vi "RT Loop message processing.vi"(7 "queue processing cycle time":u32=50 min=1 max=500, 8 "error in (no error)":errorcluster, 10 "reserved cycle for lower priority queues":u32=10 min=5 max=100) -> ()   [LabVIEW 2016]
uses:
  Globals/RT Stop.vi
  Globals/queue priority list.vi
  Message Queue/Message Queue.lvlib
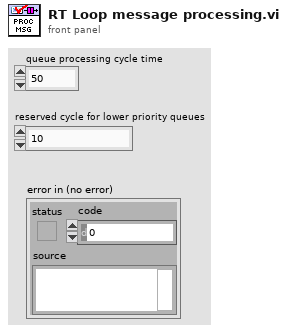
[diagram p1: front panel]
types:
  T1 = typedef "Message Queue.lvlib/queue priority list.ctl" = T2[]
  T2 = typedef "Message Queue.lvlib/queue priority info.ctl" = cluster{"queue name":string, "msg processing func ref":refnum<vi>}
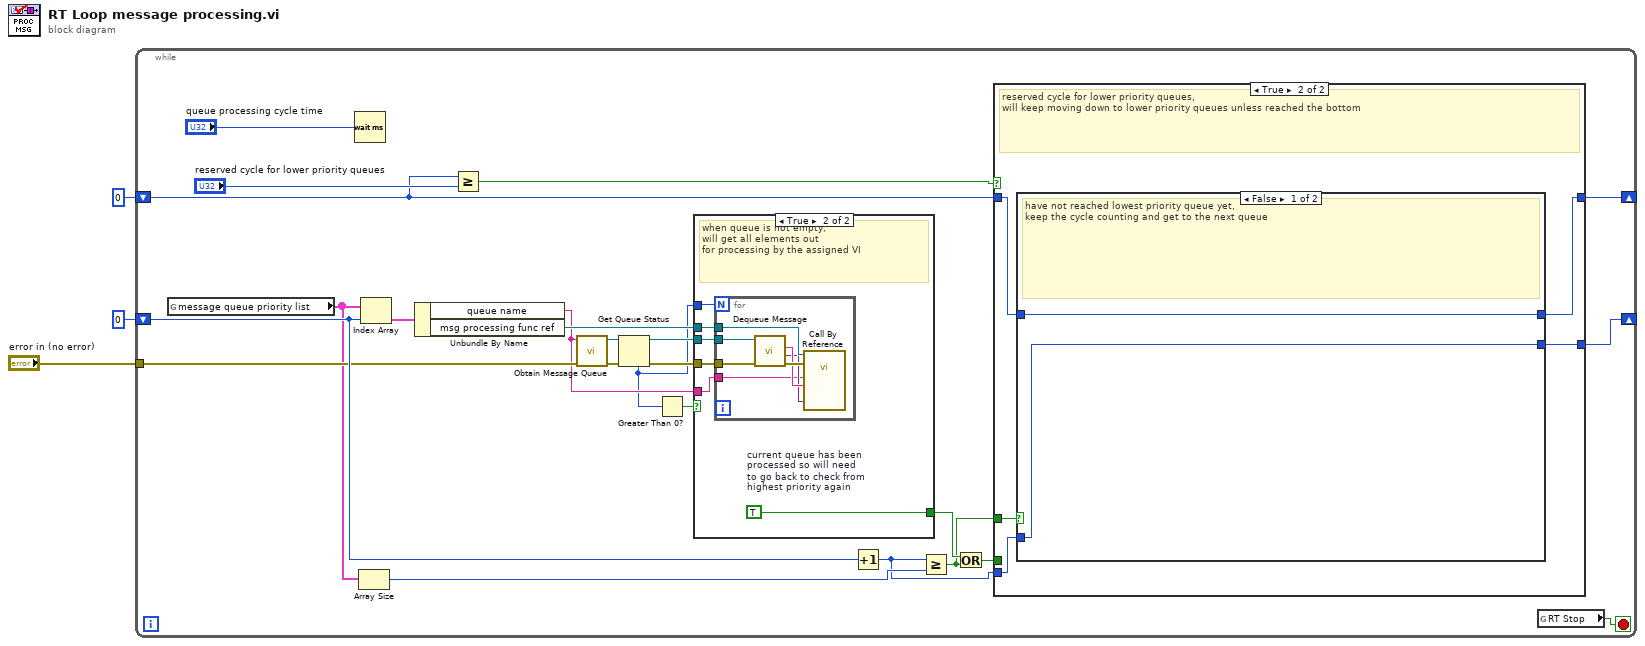
[diagram p0: block diagram]
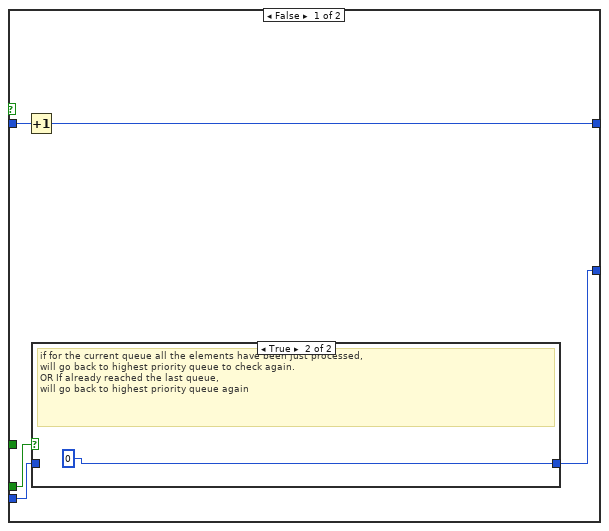
[diagram p2: hidden frame]
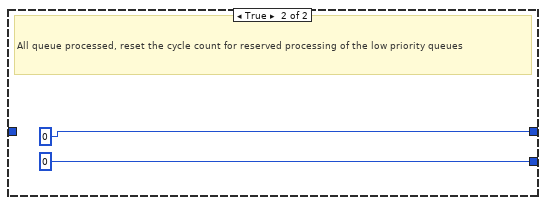
[diagram p4: hidden frame]
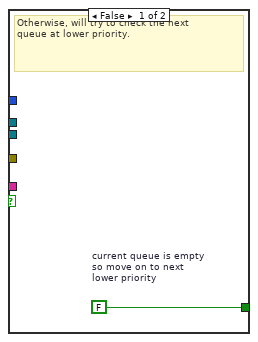
[diagram p5: hidden frame]
diagram:
  n1 = while {
    shift-right: [w24] -> _
    shift-left: 0 -> [w26]
    tunnel: "error in (no error)" -> [w25]
    shift-right: [w5] -> _
    shift-left: u32 0 -> [w6]
    stop <- w27 stop-if-true
    n2 = global read "queue priority list.vi" "message queue priority list"() -> (w16:T1)
    n3 = Wait (ms)(milliseconds to wait="queue processing cycle time") -> ()  [unwired: 1 out]
    n4 = Array Size(array=w16) -> (size(s)=w15:i32)
    n5 = Index Array(array=w16, index=w26) -> (element=w23:T2)
    n6 = Unbundle By Name(w23) -> ("queue name"=w17:string, "msg processing func ref"=w21:refnum<vi>)
    n7 = Greater Or Equal?(x=w6, y="reserved cycle for lower priority queues") -> (x >= y?=w8:bool)
    n8 = call "Obtain Message Queue.vi"("error in (no error)"=w25, "name (unnamed)"=w17) -> ("error out"=w19:errorcluster, "Message Queue"=w22:refnum<queue>)  [unwired: 7 in, 1 out]
    n9 = Get Queue Status(queue=w22, error in (no error)=w19) -> (queue out=w20:refnum<queue>, error out=w18:errorcluster, # elements in queue=w14:i32)  [unwired: 1 in, 5 out]
    n10 = Greater Than 0?(x=w14) -> (x > 0?=w13:bool)
    n11 = case shown="True" w13 {
      tunnel: w21 -> [_ w50]
      tunnel: w20 -> [_ w49]
      tunnel: w18 -> [_ w48]
      tunnel: w17 -> [_ w47]
      tunnel: w14 -> [_ w46]
      tunnel: [w44 w45] -> w11
      frame False {
        w44 = FALSE  # current queue is empty so move on to next lower priority
        # "Otherwise, will try to check the next \nqueue at lower priority."
      }
      frame True {
        w45 = TRUE  # current queue has been processed so will need to go back to check from highest priority again
        # "when queue is not empty,\nwill get all elements out\nfor processing by the assigned VI"
        n12 = for {
          N: w46 -> [_]
          tunnel: w50 -> [w57]
          tunnel: w49 -> [w56]
          tunnel: w48 -> [w55]
          tunnel: w47 -> [w51]
          n13 = call "Dequeue Message.vi"("error in (no error)"=w55, "Message Queue"=w56) -> ("error out"=w54:errorcluster, "Message Data"=w52:variant, "Message"=w53:string)  [unwired: 5 in, 2 out]
          n14 = call-by-ref "?"(reference=w57, error in=w54, "message data"=w52, "message"=w53, "message type"=w51) -> ()  [unwired: 9 in, 2 out]
        }
      }
    }
    n15 = Increment(x=w26) -> (x+1=w9:i32)
    n16 = Greater Or Equal?(x=w9, y=w15) -> (x >= y?=w7:bool)
    n17 = Or(x=w11, y=w7) -> (x .or. y?=w12:bool)
    n18 = case shown="True" w8 {
      tunnel: [w32 w38] -> w24
      tunnel: w12 -> [w31 _]
      tunnel: w9 -> [w30 w37]
      tunnel: w7 -> [_ w39]
      tunnel: w6 -> [w29 w36]
      tunnel: [w28 w35] -> w5
      frame False {
        n19 = Increment(x=w29) -> (x+1=w28:u32)
        n20 = case shown="True" w31 {
          tunnel: w30 -> [w33 _]
          tunnel: [w33 0] -> w32
          frame False {
            # "Otherwise, if the current queue has nothing in it to process, \nand there are lower priority queues,\nwill move on to the next lower priority queue\nto process messages there."
          }
          frame True {
            # "if for the current queue all the elements have been just processed,\nwill go back to highest priority queue to check again.\nOR If already reached the last queue, \nwill go back to highest priority queue again"
          }
        }
      }
      frame True {
        # "reserved cycle for lower priority queues,\nwill keep moving down to lower priority queues unless reached the bottom"
        n21 = case shown="False" w39 {
          tunnel: [w41 0] -> w38
          tunnel: w37 -> [w41 _]
          tunnel: w36 -> [w40 _]
          tunnel: [w40 u32 0] -> w35
          frame False {
            # "have not reached lowest priority queue yet,\nkeep the cycle counting and get to the next queue"
          }
          frame True {
            # "All queue processed, reset the cycle count for reserved processing of the low priority queues"
          }
        }
      }
    }
    n22 = global read "RT Stop.vi" "RT Stop"() -> (w27:bool)
  }
